vi "calibration_sub.vi"(1 "Angle in":i32, 7 "LINX Resource":T1, 8 "error in (no error)":errorcluster, 9 "DO Channels":u8[](array[numeric]), 10 "CCW":bool, 11 "Start calibration":bool) -> (0 "error out":errorcluster, 2 "LINX Resource out":T1, 3 "Actual angle out":dbl)   [LabVIEW 2020]
uses:
  <vilib>/MakerHub/LINX/Private/Type Defs/LINX Ref.ctl
  <vilib>/MakerHub/LINX/Private/Type Defs/Platform.ctl
  <vilib>/MakerHub/LINX/Private/Type Defs/Interface.ctl
  <vilib>/MakerHub/LINX/Private/Device/Type Defs/LINX Device Config.ctl
  <vilib>/MakerHub/LINX/Private/Device/Type Defs/TCP Config.ctl
  <vilib>/MakerHub/LINX/Private/Device/Type Defs/Channels.ctl
  <vilib>/MakerHub/LINX/Public/Peripherals/Digital/Digital Read 1 Chan.vi
  <vilib>/MakerHub/LINX/Public/Peripherals/Digital/Digital Read N Chans.vi
  <vilib>/MakerHub/LINX/Private/Local IO/LinxDigitalRead.vi
  <vilib>/MakerHub/LINX/Public/Utilities/Check Channel.vi
  <vilib>/MakerHub/LINX/Private/Utilties/Generate Error.vi
  <vilib>/MakerHub/LINX/LMH-LINX.lvlib
  <vilib>/MakerHub/LINX/Private/Device/Device.lvlib
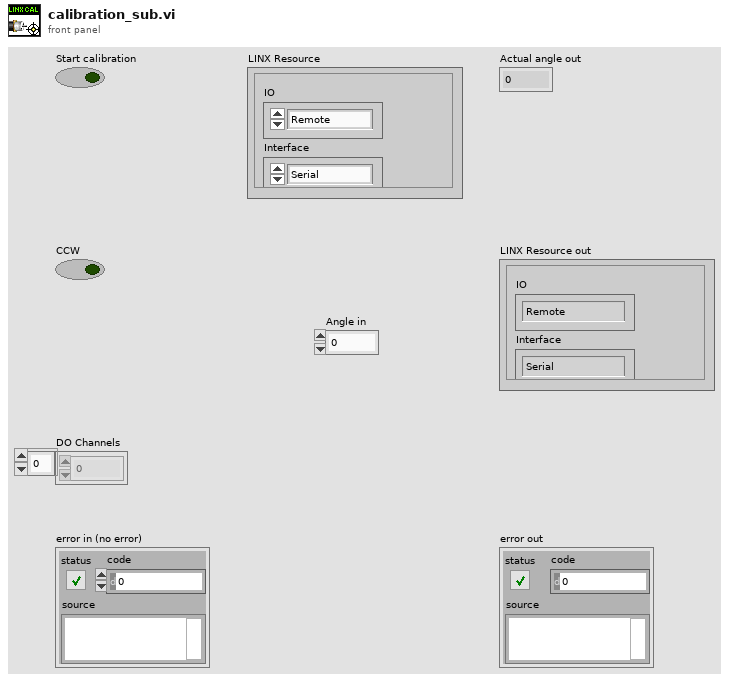
[diagram p1: front panel]
types:
  T1 = typedef "LMH-LINX.lvlib/LINX Ref.ctl" = cluster{"IO":T2, "Interface":T3, "LINX Device Config":T4}
  T2 = typedef "LMH-LINX.lvlib/Platform.ctl" = enum16{"Remote", "Local"}
  T3 = typedef "LMH-LINX.lvlib/Interface.ctl" = enum16{"Serial", "TCP"}
  T4 = typedef "LMH-LINX.lvlib/Device.lvlib/LINX Device Config.ctl" = cluster{"Interface":T3, "COM Port":refnum<visa-resource-name>, "TCP Configuration":T5, "Device Family":u8, "Device ID":u8, "Device Name":string, "TCP Ref":refnum<k5>, "Channels":T6}
  T5 = typedef "LMH-LINX.lvlib/Device.lvlib/TCP Config.ctl" = cluster{"IP Address":string, "Port":u16}
  T6 = typedef "LMH-LINX.lvlib/Channels.ctl" = cluster{"DI":u8[], "DO":u8[], "AI":u8[], "AO":u8[], "PWM":u8[], "QE":u8[], "UART":u8[], "I2C 2":u8[], "SPI":u8[], "CAN":u8[], "Servo":u8[], "AI Ref (V)":dbl, "AI Resolution (Bits)":u8, "AO Ref (V)":dbl, "AO Resolution (Bits)":u8}
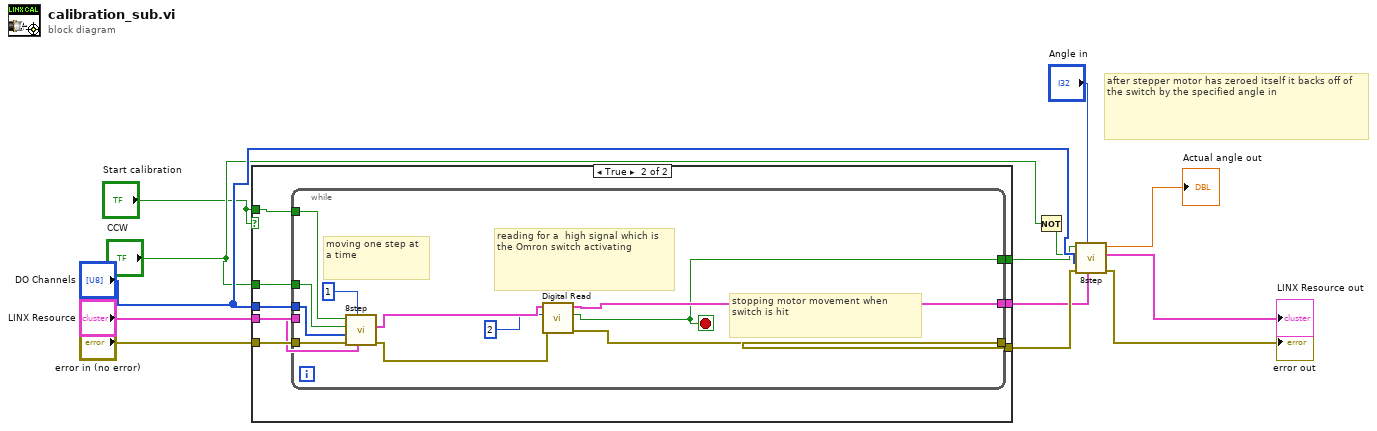
[diagram p0: block diagram]
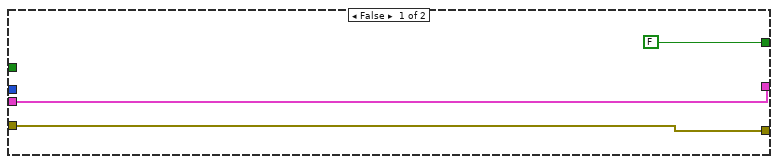
[diagram p2: hidden frame]
diagram:
  # "after stepper motor has zeroed itself it backs off of the switch by the specified angle in"
  n1 = case shown="True" "Start calibration" {
    tunnel: "Start calibration" -> [_ w24]
    tunnel: "LINX Resource" -> [w16 w23]
    tunnel: "error in (no error)" -> [w15 w22]
    tunnel: "DO Channels" -> [_ w21]
    tunnel: "CCW" -> [_ w20]
    tunnel: [w16 w19] -> w5
    tunnel: [w15 w18] -> w6
    tunnel: [FALSE w17] -> w9
    frame False {
    }
    frame True {
      n2 = while {
        tunnel: w24 -> [w36]
        tunnel: w21 -> [w33]
        tunnel: w20 -> [w26]
        tunnel: w22 -> [w34]
        tunnel: w23 -> [w35]
        tunnel: [w30] -> w19
        tunnel: [w27] -> w18
        tunnel: [w25] -> w17
        stop <- w25 stop-if-true
        # "stopping motor movement when switch is hit"
        # "moving one step at a time"
        # "reading for a  high signal which is the Omron switch activating"
        n3 = call "8step.vi"("LINX Resource in"=w35, "Angle in"=1, "error in (no error)"=w34, "DO Channels"=w33, "CCW"=w26, "OK Button"=w36) -> ("error out"=w28:errorcluster, "LINX Resource out"=w31:T1)  [unwired: 3 in, 1 out]
        n4 = call-poly <vilib>:"Digital Read.vi"("Error In"=w28, "DI Channel"=u8 2 ("Analog Channel"), "LINX Resource"=w31) -> ("Error Out"=w27:errorcluster, "DI Value"=w25:bool, "LINX Resource"=w30:T1)  [unwired: 6 in]
      }
    }
  }
  n5 = Not(x="CCW") -> (.not. x?=w11:bool)
  n6 = call "8step.vi"("LINX Resource in"=w5, "Angle in"="Angle in", "error in (no error)"=w6, "DO Channels"="DO Channels", "CCW"=w11, "OK Button"=w9) -> ("error out"=→"error out":errorcluster, "LINX Resource out"=→"LINX Resource out":T1, "Actual angle out"=→"Actual angle out":dbl)  [unwired: 3 in]
